vi "OnOperateClick.vi"(0 "XRef":T15, 1 "Point":T13, 2 "State In":T1) -> (14 "Reply":T11, 15 "Fatal Error Out":T10, 16 "State Out":T1)   [LabVIEW 2020, in "FlexBlock.xnode"]
uses:
  FlexBlock.xnode
  <vilib>/XNodeSupport/XNodeXNodeRef.ctl
  <vilib>/XNodeSupport/XNodePoint.ctl
  <vilib>/XNodeSupport/XNodeInt.ctl
  State.ctl
  FlexBlocks/Type Descriptor.ctl
  FlexBlocks/Terminal Direction.ctl
  FlexBlocks/Value Mode.ctl
  FlexBlocks/Terminal State.ctl
  FlexBlocks/Special Terminal.ctl
  FlexBlocks/Errors.ctl
  <vilib>/picture/picture.llb/imagedata.ctl
  FlexBlocks/Calculated Sizes.ctl
  <vilib>/XNodeSupport/XNodeStringArray.ctl
  <vilib>/XNodeSupport/XNodeString.ctl
  <vilib>/XNodeSupport/XNodeErrorCluster.ctl
  <vilib>/XNodeSupport/NI_XNodeSupport.lvlib
  FlexBlocks/FlexBlocks.lvlib
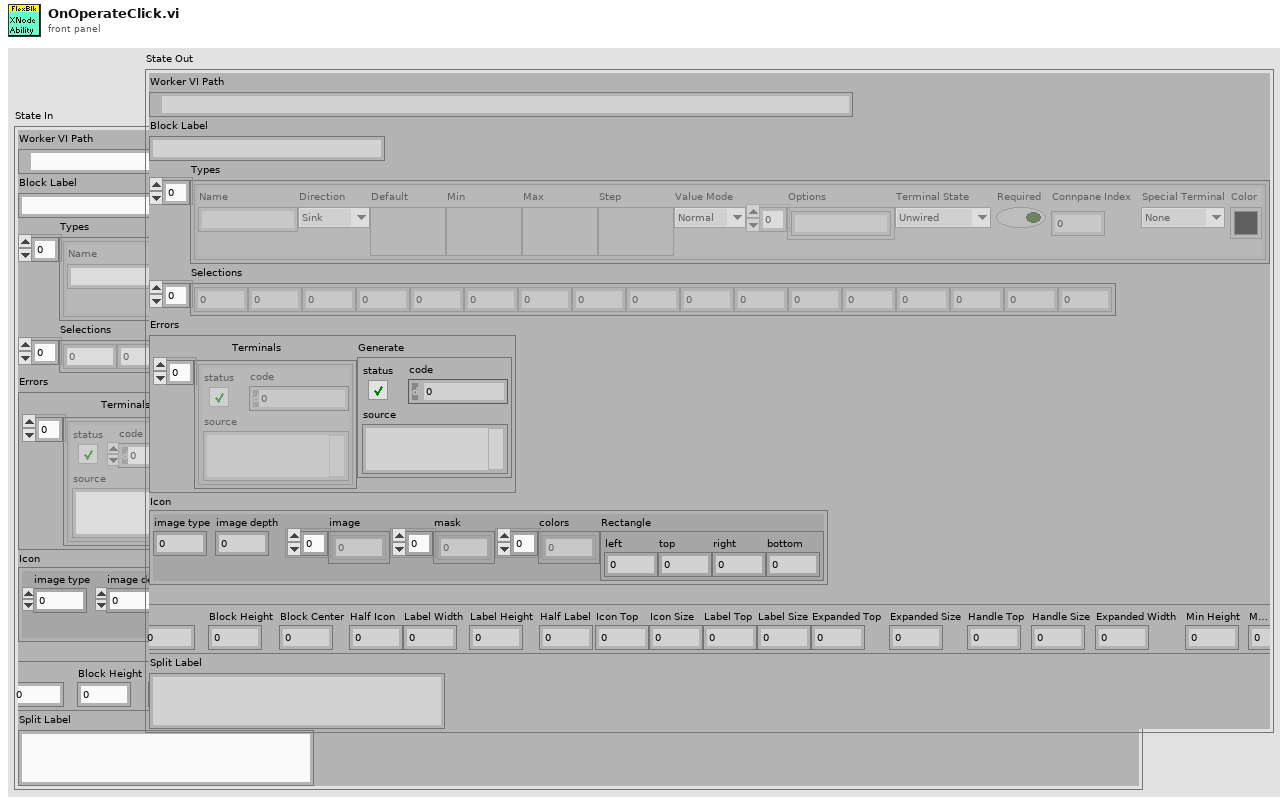
[diagram p1: front panel]
types:
  T1 = typedef "FlexBlock.xnode/State.ctl" = cluster{"Worker VI Path":path, "Block Label":string, "Types":T2[], "Selections":i32[], "Errors":T7, "Icon":T8, "Calcd Sizes":T9, "Split Label":string}
  T2 = typedef "FlexBlocks.lvlib/Type Descriptor.ctl" = cluster{"Name":string, "Direction":T3, "Default":variant, "Min":variant, "Max":variant, "Step":variant, "Value Mode":T4, "Options":string[], "Terminal State":T5, "Required":bool, "Connpane Index":i32, "Special Terminal":T6, "Color":u32}
  T3 = typedef "FlexBlocks.lvlib/Terminal Direction.ctl" = enum16{"Sink", "Source"}
  T4 = typedef "FlexBlocks.lvlib/Value Mode.ctl" = enum16{"Normal", "Range", "Select"}
  T5 = typedef "FlexBlocks.lvlib/Terminal State.ctl" = enum16{"Unwired", "BadType", "BadRef", "Channel", "Value", "Control Ref"}
  T6 = typedef "FlexBlocks.lvlib/Special Terminal.ctl" = enum16{"None", "Action", "Init", "Tag", "State in", "State out", "Error"}
  T7 = typedef "FlexBlocks.lvlib/Errors.ctl" = cluster{"Terminals":errorcluster[], "Generate":errorcluster}
  T8 = typedef "imagedata.ctl" = cluster{"image type":i32, "image depth":i32, "image":u8[], "mask":u8[], "colors":u32[], "Rectangle":cluster{"left":i16, "top":i16, "right":i16, "bottom":i16}}
  T9 = typedef "FlexBlocks.lvlib/Calculated Sizes.ctl" = cluster{"Text Width":i32, "Text Height":i32, "Half Text":i32, "Block Width":i32, "Block Height":i32, "Block Center":i32, "Half Icon":i32, "Label Width":i32, "Label Height":i32, "Half Label":i32, "Icon Top":i32, "Icon Size":i32, "Label Top":i32, "Label Size":i32, "Expanded Top":i32, "Expanded Size":i32, "Handle Top":i32, "Handle Size":i32, "Expanded Width":i32, "Min Height":i32, "Max Height":i32}
  T10 = typedef "NI_XNodeSupport.lvlib/XNodeErrorCluster.ctl" = errorcluster
  T11 = typedef "NI_XNodeSupport.lvlib/XNodeStringArray.ctl" = T12[]
  T12 = typedef "NI_XNodeSupport.lvlib/XNodeString.ctl" = string
  T13 = typedef "NI_XNodeSupport.lvlib/XNodePoint.ctl" = cluster{"H":T14, "V":T14}
  T14 = typedef "NI_XNodeSupport.lvlib/XNodeInt.ctl" = i32
  T15 = typedef "NI_XNodeSupport.lvlib/XNodeXNodeRef.ctl" = refnum<vi>
  T16 = cluster{"left":i16, "top":i16, "right":i16, "bottom":i16}
  T17 = typedef "FlexBlocks.lvlib/Size Constants.ctl" = cluster{"Icon":i32, "Value Width":i32, "BG Rounding":i32, "Term Width":i32, "Term Height":i32, "Text Offset":i32, "Value Padding":i32, "Select Padding":i32, "Min Block Width":i32, "Vertical Margin":i32, "Size Handle Height":i32, "Name Padding":i32, "Collapsed Spacing":i32}
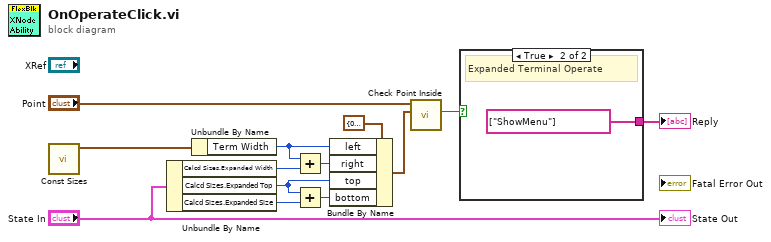
[diagram p0: block diagram]
diagram:
  n1 = call "Const Sizes.vi"() -> ("Sizes"=w1:T17)  [unwired: 11 in]
  n2 = Unbundle By Name("State In") -> ("Calcd Sizes.Expanded Width"=w10:i32, "Calcd Sizes.Expanded Top"=w7:i32, "Calcd Sizes.Expanded Size"=w8:i32)
  n3 = Unbundle By Name(w1) -> ("Term Width"=w9:i32)
  n4 = Add(x=w9, y=w10) -> (x+y=w11:i32)
  n5 = Add(x=w7, y=w8) -> (x+y=w6:i32)
  n6 = Bundle By Name(cluster=T16 {"left"=0, "top"=0, "right"=0, "bottom"=0} ("rect"), "left"=w9, "right"=w11, "top"=w7, "bottom"=w6) -> (w4:T16)
  n7 = call "Check Point Inside.vi"("rect"=w4, "Point In"="Point") -> ("Inside"=w5:bool)  [unwired: 8 in, 1 out]
  n8 = case shown="True" w5 {
    tunnel: [_ T11 ["ShowMenu"] ("Reply")] -> w2
    frame False {
      # "Outside Expanded Terminals"
    }
    frame True {
      # "Expanded Terminal Operate"
    }
  }
  "Reply" <- w2
  "State Out" <- "State In"
